vi "queue.vi"(0 "Input":i32, 9 "Enum":T1, 11 "error in":errorcluster) -> (4 "Output":i32, 10 "Array":i32[](array[numeric]), 15 "error out":errorcluster)   [LabVIEW 2023]
uses:
  queue_op.ctl
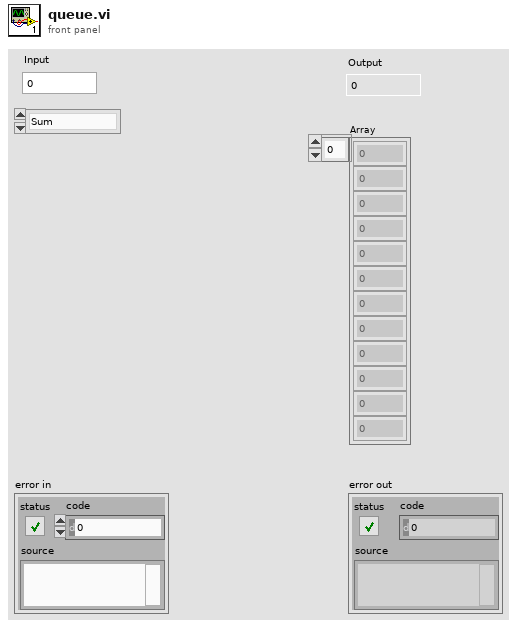
[diagram p1: front panel]
types:
  T1 = typedef "queue_op.ctl" = enum16{"Sum", "Dequeue", "Enqueue", "Initialize"}
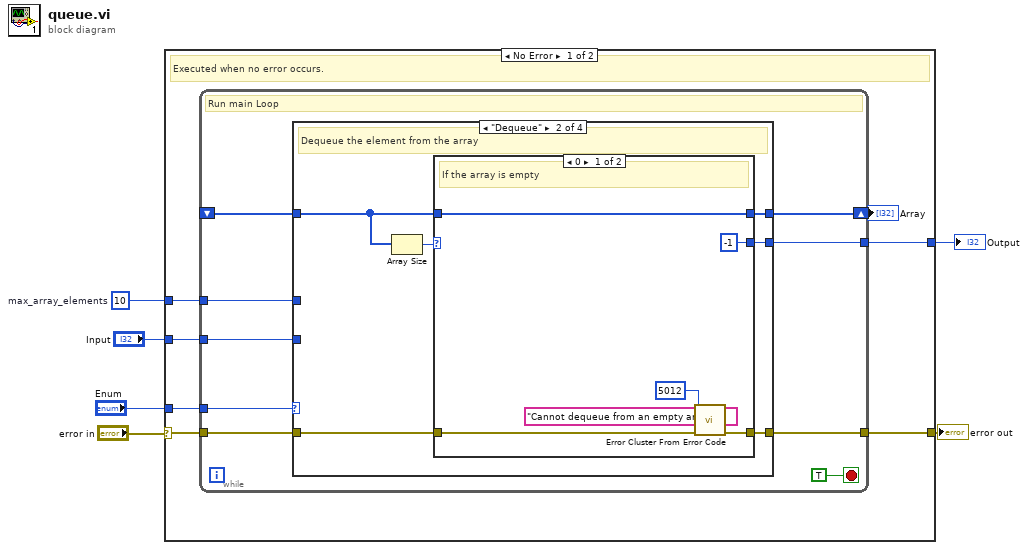
[diagram p0: block diagram]
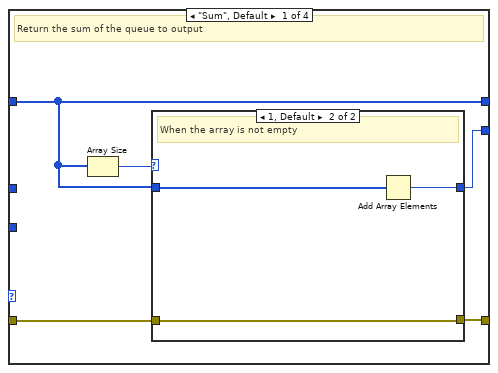
[diagram p2: hidden frame]
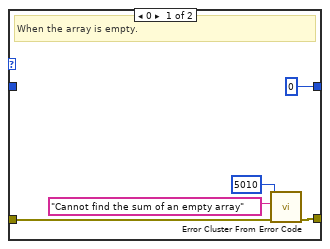
[diagram p3: hidden frame]
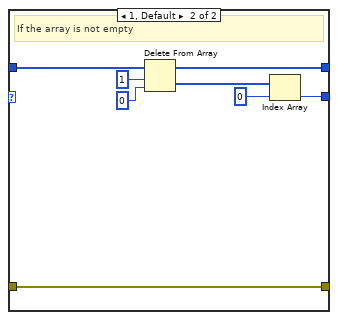
[diagram p4: hidden frame]
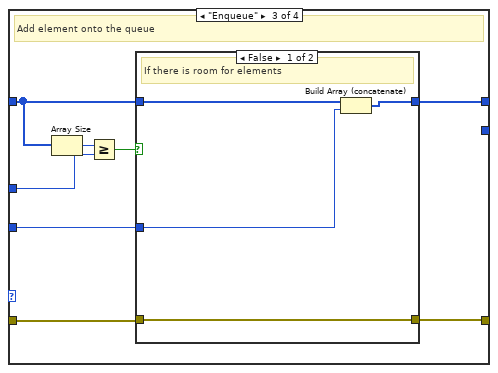
[diagram p5: hidden frame]
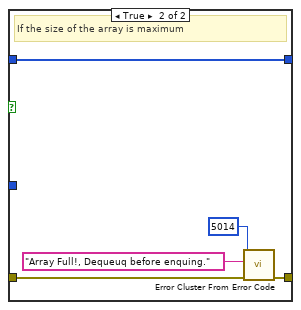
[diagram p6: hidden frame]
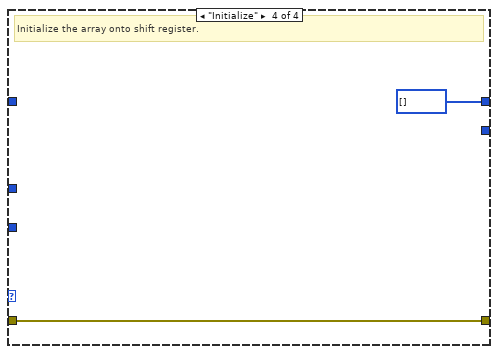
[diagram p7: hidden frame]
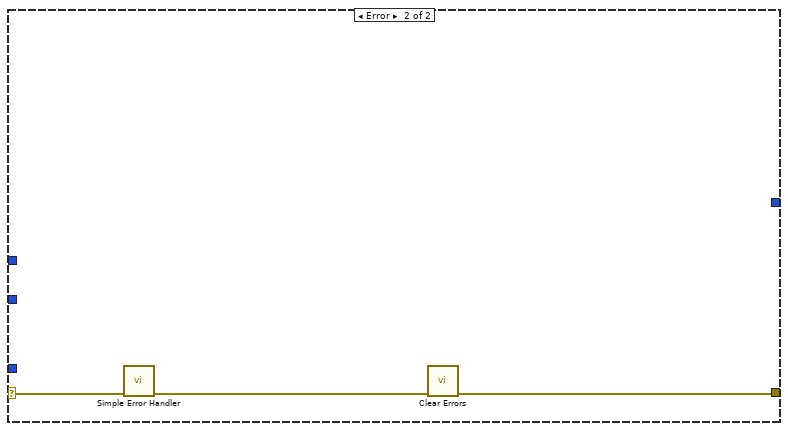
[diagram p8: hidden frame]
diagram:
  w1 = 10  # max_array_elements
  n1 = case shown="No Error" "error in" {
    selector: "error in" -> [w12 w77]
    tunnel: [w13 w75] -> w5
    tunnel: "Enum" -> [w11 _]
    tunnel: "Input" -> [w10 _]
    tunnel: [w9 _] -> w2
    tunnel: w1 -> [w7 _]
    frame No Error {
      # "Executed when no error occurs."
      n2 = while {
        tunnel: [w21] -> w13
        tunnel: w12 -> [w20]
        shift-right: [w17] -> w8
        shift-left: _ -> [w18]
        tunnel: w11 -> [w19]
        tunnel: w10 -> [w16]
        tunnel: [w15] -> w9
        tunnel: w7 -> [w14]
        stop <- TRUE stop-if-true
        # "Run main Loop"
        n3 = case shown="\"Dequeue\"" w19 {
          tunnel: [w26 w36 w57 w74] -> w21
          tunnel: w20 -> [w27 w37 w56 w74]
          tunnel: w18 -> [w24 w40 w60 _]
          tunnel: [w24 w41 w62 i32[] []] -> w17
          tunnel: w16 -> [_ _ w63 _]
          tunnel: [w23 w38 _ _] -> w15
          tunnel: w14 -> [_ _ w59 _]
          frame "Sum", Default {
            # "Return the sum of the queue to output"
            n4 = Array Size(array=w24) -> (size(s)=w25:i32)
            n5 = case shown="1, Default" w25 {
              tunnel: [w31 w35] -> w26
              tunnel: w27 -> [w32 w35]
              tunnel: w24 -> [_ w34]
              tunnel: [0 ("Input") w33] -> w23
              frame 0 {
                # "When the array is empty."
                n6 = call <vilib>:"Error Cluster From Error Code.vi"("error in (no error)"=w32, "error message (\"\")"="Cannot find the sum of an empty array" ("error message (\"\")"), "error code (0)"=5010) -> ("error out"=w31:errorcluster)  [unwired: 6 in]
              }
              frame 1, Default {
                # "When the array is not empty"
                n7 = Add Array Elements(numeric array=w34) -> (sum=w33:i32)
              }
            }
          }
          frame "Dequeue" {
            # "Dequeue the element from the array"
            n8 = Array Size(array=w40) -> (size(s)=w39:i32)
            n9 = case shown="0" w39 {
              tunnel: [w47 w55] -> w41
              tunnel: w40 -> [w47 w53]
              tunnel: [-1 ("Input") w50] -> w38
              tunnel: w37 -> [w44 w49]
              tunnel: [w45 w49] -> w36
              frame 0 {
                # "If the array is empty"
                n10 = call <vilib>:"Error Cluster From Error Code.vi"("error in (no error)"=w44, "error message (\"\")"="Cannot dequeue from an empty array !" ("error message (\"\")"), "error code (0)"=5012) -> ("error out"=w45:errorcluster)  [unwired: 6 in]
              }
              frame 1, Default {
                # "If the array is not empty"
                n11 = Delete From Array(array=w53, length=1, index=0) -> (deleted portion=w52:i32[], array with subset deleted=w55:i32[])
                n12 = Index Array(array=w52, index=0) -> (element=w50:i32)
              }
            }
          }
          frame "Enqueue" {
            # "Add element onto the queue"
            n13 = Array Size(array=w60) -> (size(s)=w61:i32)
            n14 = Greater Or Equal?(x=w61, y=w59) -> (x >= y?=w58:bool)
            n15 = case shown="False" w58 {
              tunnel: w60 -> [w67 w71]
              tunnel: w63 -> [w66 _]
              tunnel: [w65 w71] -> w62
              tunnel: [w64 w70] -> w57
              tunnel: w56 -> [w64 w72]
              frame False {
                # "If there is room for elements"
                n16 = Build Array (concatenate)(w67, w66) -> (w65:i32[])
              }
              frame True {
                # "If the size of the array is maximum"
                n17 = call <vilib>:"Error Cluster From Error Code.vi"("error in (no error)"=w72, "error message (\"\")"="Array Full!, Dequeuq before enquing." ("error message (\"\")"), "error code (0)"=5014) -> ("error out"=w70:errorcluster)  [unwired: 6 in]
              }
            }
          }
          frame "Initialize" {
            # "Initialize the array onto shift register."
          }
        }
      }
      "Array" <- w8
    }
    frame Error {
      n18 = call <vilib>:"Simple Error Handler.vi"("error in (no error)"=w77) -> ("error out"=w76:errorcluster)  [unwired: 4 in, 4 out]
      n19 = call <vilib>:"Clear Errors.vi"("error in (no error)"=w76) -> ("error out"=w75:errorcluster)  [unwired: 5 in, 1 out]
    }
  }
  "Output" <- w2
  "error out" <- w5
